vi "START RETURN ITEMS.vi"(11 "REFERENCES":T1) -> ()   [LabVIEW 2019]
uses:
  Controls/References Cluster.ctl
  Controls/Custom Calendar/Custom Calendar.xctl
  Controls/Column Names/Inventory Column Names.ctl
  <vilib>/Utility/miscctls.llb/LVRowAndColumnTypeDef.ctl
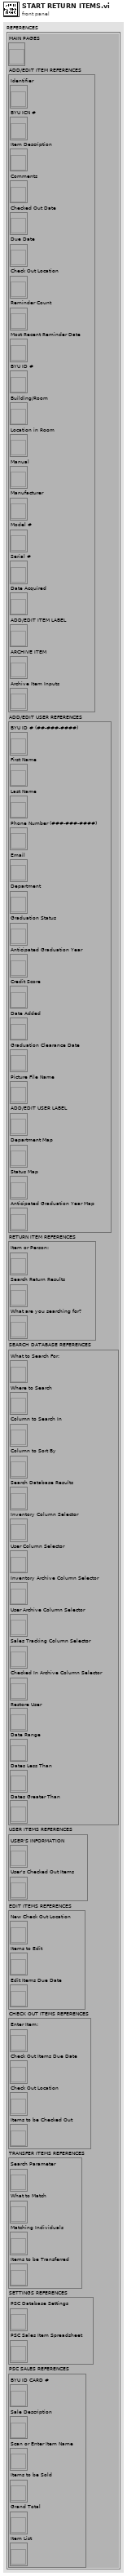
[diagram p1: front panel]
types:
  T1 = typedef "References Cluster.ctl" = cluster{"MAIN PAGES":refnum<vi>, "ADD/EDIT ITEM REFERENCES":cluster{"Identifier":refnum<vi>, "BYU ICN #":refnum<vi>, "Item Description":refnum<vi>, "Comments":refnum<vi>, "Checked Out Date":refnum<vi>, "Due Date":refnum<vi>, "Check Out Location":refnum<vi>, "Reminder Count":refnum<vi>, "Most Recent Reminder Date":refnum<vi>, "BYU ID #":refnum<vi>, "Building/Room":refnum<vi>, "Location in Room":refnum<vi>, "Manual":refnum<vi>, "Manufacturer":refnum<vi>, "Model #":refnum<vi>, "Serial #":refnum<vi>, "Date Acquired":refnum<vi>, "ADD/EDIT ITEM LABEL":refnum<vi>, "ARCHIVE ITEM":refnum<vi>, "Archive Item Inputs":refnum<vi>}, "ADD/EDIT USER REFERENCES":cluster{"BYU ID # (##-###-####)":refnum<vi>, "First Name":refnum<vi>, "Last Name":refnum<vi>, "Phone Number (###-###-####)":refnum<vi>, "Email":refnum<vi>, "Department":refnum<vi>, "Graduation Status":refnum<vi>, "Anticipated Graduation Year":refnum<vi>, "Credit Score":refnum<vi>, "Date Added":refnum<vi>, "Graduation Clearance Date":refnum<vi>, "Picture File Name":refnum<vi>, "ADD/EDIT USER LABEL":refnum<vi>, "Department Map":refnum<vi>, "Status Map":refnum<vi>, "Anticipated Graduation Year Map":refnum<vi>}, "RETURN ITEM REFERENCES":cluster{"Item or Person:":refnum<vi>, "Search Return Results":refnum<vi>, "What are you searching for?":refnum<vi>}, "SEARCH DATABASE REFERENCES":cluster{"What to Search For:":refnum<vi>, "Where to Search":refnum<vi>, "Column to Search In":refnum<vi>, "Column to Sort By":refnum<vi>, "Search Database Results":refnum<vi>, "Inventory Column Selector":refnum<vi>, "User Column Selector":refnum<vi>, "Inventory Archive Column Selector":refnum<vi>, "User Archive Column Selector":refnum<vi>, "Sales Tracking Column Selector":refnum<vi>, "Checked In Archive Column Selector":refnum<vi>, "Restore User":refnum<vi>, "Date Range":refnum<vi>, "Dates Less Than":refnum<vi>, "Dates Greater Than":refnum<vi>}, "USER ITEMS REFERENCES":cluster{"USER'S INFORMATION":refnum<vi>, "User's Checked Out Items":refnum<vi>}, "EDIT ITEMS REFERENCES":cluster{"New Check Out Location":refnum<vi>, "Items to Edit":refnum<vi>, "Edit Items Due Date":refnum<vi>}, "CHECK OUT ITEMS REFERENCES":cluster{"Enter Item:":refnum<vi>, "Check Out Items Due Date":refnum<vi>, "Check Out Location":refnum<vi>, "Items to be Checked Out":refnum<vi>}, "TRANSFER ITEMS REFERENCES":cluster{"Search Parameter":refnum<vi>, "What to Match":refnum<vi>, "Matching Individuals":refnum<vi>, "Items to be Transferred":refnum<vi>}, "SETTINGS REFERENCES":cluster{"PSC Database Settings":refnum<vi>, "PSC Sales Item Spreadsheet":refnum<vi>}, "PSC SALES REFERENCES":cluster{"BYU ID CARD #":refnum<vi>, "Sale Description":refnum<vi>, "Scan or Enter Item Name":refnum<vi>, "Items to be Sold":refnum<vi>, "Grand Total":refnum<vi>, "Item List":refnum<vi>}}
  T2 = typedef "LVRowAndColumnTypeDef.ctl" = cluster{"Row":i32, "Column":i32}
  T3 = typedef "Inventory Column Names.ctl" = string[]
  T4 = enum32{"IDLE", "ADD/EDIT USER", "ADD/EDIT ITEM", "RETURN ITEMS", "SEARCH DATABASE", "USER ITEMS", "CHECK OUT ITEMS", "EDIT ITEMS", "TRANSFER ITEMS", "PSC SALES", "ATRIUM", "INVENTORY TRACKING", "SETTINGS"}
  T5 = cluster{"Item or Person:":refnum<vi>, "Search Return Results":refnum<vi>, "What are you searching for?":refnum<vi>}
  T6 = cluster{"Font Name:":string, "Size":i16, "Strikeout?":bool, "Italic?":bool, "Underline?":bool, "Outline?":bool, "Shadow?":bool, "Bold?":bool}
  T7 = cluster{"horizontal":enum16{"left", "center", "right"}, "vertical":enum16{"top", "center", "bottom"}}
  T8 = enum16{"User-specified Font", "Application Font", "System Font", "Dialog Font"}
  T9 = cluster{"left":i16, "top":i16, "right":i16, "bottom":i16}
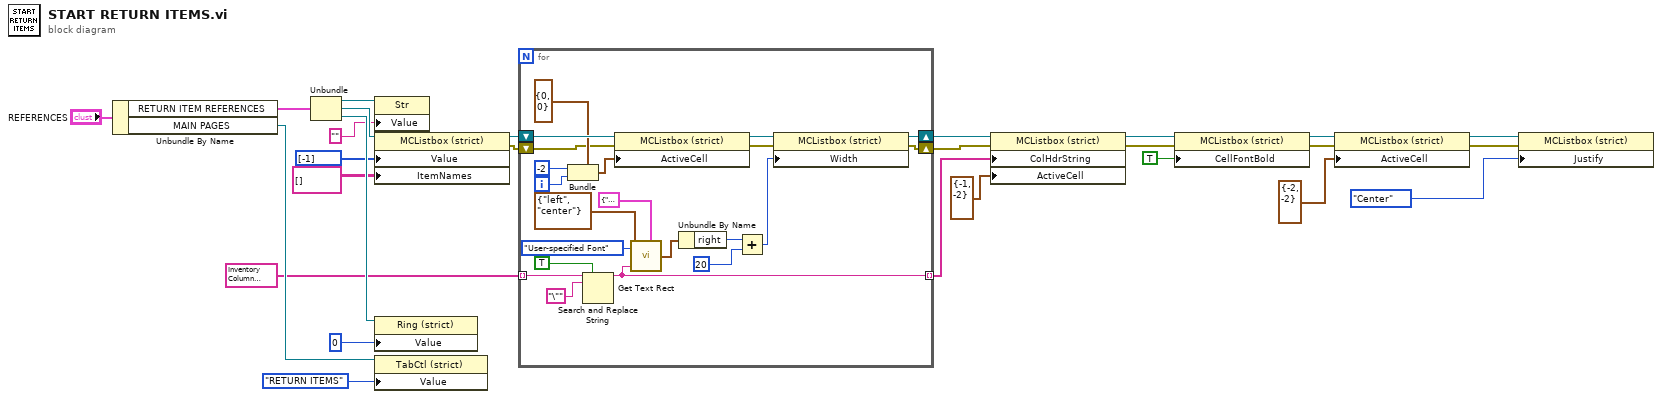
[diagram p0: block diagram]
diagram:
  n1 = Unbundle By Name("REFERENCES") -> ("RETURN ITEM REFERENCES"=w19:T5, "MAIN PAGES"=w18:refnum<vi>)
  n2 = Unbundle(w19) -> ("Item or Person:"=w27:refnum<vi>, "Search Return Results"=w26:refnum<vi>, "What are you searching for?"=w25:refnum<vi>)
  n3 = property class="Str"(reference=w27, "Value"="") -> ()  [unwired: 1 in, 2 out]
  n4 = property class="MCListbox (strict)"(reference=w26, "Value"=i32[] [-1], "ItemNames"=string[][] [] ("Item Names")) -> (reference out=w16:refnum<vi>, error out=w14:errorcluster)  [unwired: 1 in]
  n5 = property class="Ring (strict)"(reference=w25, "Value"=u16 0) -> ()  [unwired: 1 in, 2 out]
  n6 = property class="TabCtl (strict)"(reference=w18, "Value"=T4."RETURN ITEMS") -> ()  [unwired: 1 in, 2 out]
  n7 = for {
    tunnel: T3 ["\"Identifier\"", "\"BYU ICN #\"", "\"Item Description\"", "\"Comments\"", "\"Checked Out Date\"", "\"Due Date\"", "\"Check Out Location\"", "\"Reminder Count\"", "\"Most Recent Reminder Date\"", "\"BYU ID #\"", "\"Building/Room\"", "\"Location in Room\"", "\"Manual\"", "\"Manufacturer\"", "\"Model #\"", "\"Serial #\"", "\"Date Acquired\""] ("INVENTORY COLUMN NAMES") -> [w36] mode=indexing
    shift-right: [w40] -> w13
    shift-left: w16 -> [w48]
    shift-right: [w37] -> w12
    shift-left: w14 -> [w39]
    tunnel: [w32] -> w11 mode=indexing
    i -> [w45]
    n8 = Bundle(cluster=T2 {"Row"=0, "Column"=0} ("Active Cell:Active Cell"), "Row"=-2, "Column"=w45) -> (w44:T2)
    n9 = Search and Replace String(replace all?=TRUE ("replace all? (F)"), input string=w36, search string="\"") -> (result string=w32:string)  [unwired: 5 in, 3 out]
    n10 = property class="MCListbox (strict)"(reference=w48, error in=w39, "ActiveCell"=w44) -> (reference out=w41:refnum<vi>, error out=w38:errorcluster)
    n11 = call <vilib>:"Get Text Rect.vi"("alignment(left, top)"=T7 {"horizontal"=enum."left", "vertical"=enum."center"}, "desired font(Application)"=T8."User-specified Font", "text"=w32, "[user-specified font]"=T6 {"Font Name:"="", "Size"=15, "Strikeout?"=FALSE, "Italic?"=FALSE, "Underline?"=FALSE, "Outline?"=FALSE, "Shadow?"=FALSE, "Bold?"=TRUE}) -> ("rect"=w42:T9)  [unwired: 5 in]
    n12 = Unbundle By Name(w42) -> ("right"=w31:i16)
    n13 = Add(x=w31, y=i16 20) -> (x+y=w29:i16)
    n14 = property class="MCListbox (strict)"(reference=w41, error in=w38, "Width"=w29) -> (reference out=w40:refnum<vi>, error out=w37:errorcluster)
  }
  n15 = property class="MCListbox (strict)"(reference=w13, error in=w12, "ColHdrString"=w11, "ActiveCell"=T2 {"Row"=-1, "Column"=-2} ("Active Cell:Active Cell")) -> (reference out=w9:refnum<vi>, error out=w8:errorcluster)
  n16 = property class="MCListbox (strict)"(reference=w9, error in=w8, "CellFontBold"=TRUE ("Active Cell:Cell Font:Bold")) -> (reference out=w6:refnum<vi>, error out=w5:errorcluster)
  n17 = property class="MCListbox (strict)"(reference=w6, error in=w5, "ActiveCell"=T2 {"Row"=-2, "Column"=-2} ("Active Cell:Active Cell")) -> (reference out=w3:refnum<vi>, error out=w2:errorcluster)
  n18 = property class="MCListbox (strict)"(reference=w3, error in=w2, "Justify"=enum16{"Left", "Center", "Right"}."Center" ("Active Cell:Cell Justification")) -> ()  [unwired: 2 out]
